vi "FTW-STR-Explode.vi"(0 "Input String":string, 5 "Regex Delimiter (,)":string=",", 11 "error in":errorcluster) -> (4 "Pieces":string[](array[string]), 15 "error out":errorcluster)   [LabVIEW 2015]
doc: "Creates an array of strings by splitting a string into pieces based on a delimiter. Leading and trailing delimiters are ignored. Consecutive repeat delimiters are treated as a single delimter."
uses:
  regex/FTW-Regex-Execute.vi
  error/FTW-ERR-ThrowGenericError.vi
  error/FTW-ERR-ThrowError.vi
  error/FTW-ERR-CallChain.vi
  error/FTW-ERR-NoErrorConstant.vi
  FTW-STR-ReplaceWhitespace.vi
  FTW-STR-Array-Delimit.vi
  regex/FTW-Regex-Construct.vi
  lib/FTW-KernelFilepath.vi
  regex/FTW-Regex-Destroy.vi
panel:
  # "Inputs"
  # "Outputs"
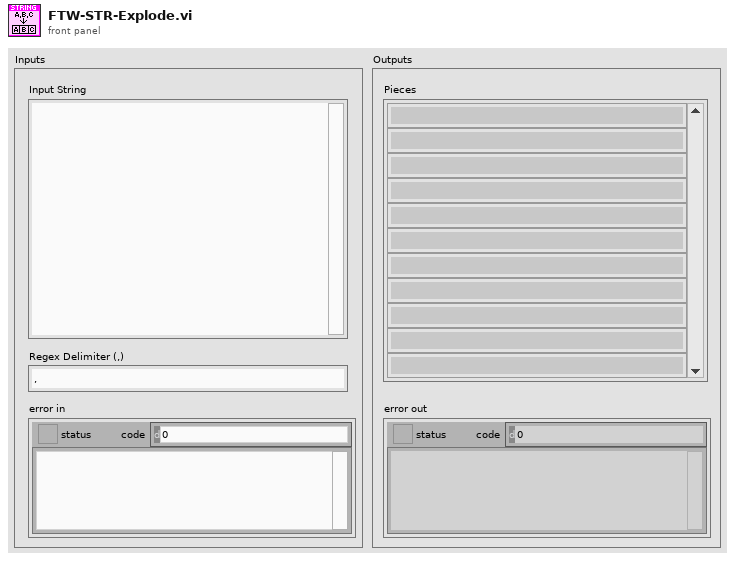
[diagram p1: front panel]
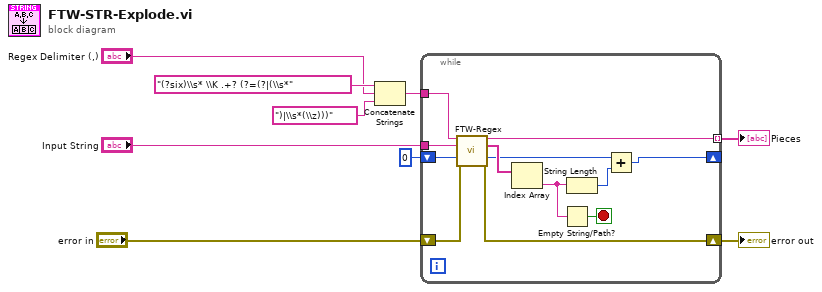
[diagram p0: block diagram]
diagram:
  n1 = Concatenate Strings("(?six)\\s* \\K .+? (?=(?|(\\s*", "Regex Delimiter (,)", ")|\\s*(\\z)))") -> (w6:string)
  n2 = while {
    tunnel: "Input String" -> [w21]
    shift-right: [w12] -> _
    shift-left: 0 ("Offset after Match") -> [w18]
    shift-right: [w19] -> w2
    shift-left: "error in" -> [w20]
    tunnel: w6 -> [w17]
    tunnel: [w16] -> w4 mode=indexing
    stop <- w10 stop-if-true
    n3 = call "FTW-Regex.vi"("Regular Expression"=w17, "Input String"=w21, "Starting Offset"=w18, "error in"=w20) -> ("Match"=w16:string, "Submatches"=w15:string[], "Offset after Match"=w13:i32, "error out"=w19:errorcluster)  [unwired: 7 in, 1 out]
    n4 = Index Array(array=w15) -> (element=w11:string)  [unwired: 1 in]
    n5 = Empty String/Path?(string/path=w11) -> (empty?=w10:bool)
    n6 = String Length(string=w11) -> (length=w14:i32)
    n7 = Add(x=w13, y=w14) -> (x+y=w12:i32)
  }
  "Pieces" <- w4
  "error out" <- w2
